vi "Goal Classifier.vi"(5 "ResolutionY":dbl, 7 "ResolutionX":dbl, 11 "InArray":dbl[][](array[numeric])) -> (3 "OutArray":dbl[][](array[numeric]))   [LabVIEW 2012]
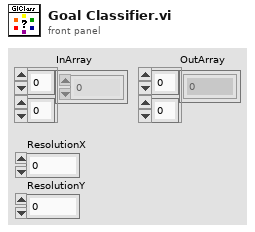
[diagram p1: front panel]
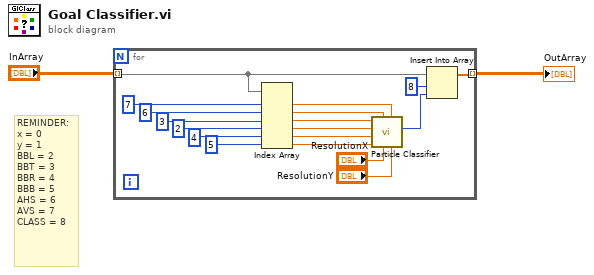
[diagram p0: block diagram]
diagram:
  # "REMINDER:\nx = 0\ny = 1\nBBL = 2\nBBT = 3\nBBR = 4 \nBBB = 5 \nAHS = 6\nAVS = 7 \nCLASS = 8"
  n1 = for {
    tunnel: "InArray" -> [w14] mode=indexing
    tunnel: [w12] -> w1 mode=indexing
    n2 = Index Array(array=w14, index #1=7 ("index"), index #2=6 ("index"), index #3=3 ("index"), index #4=2 ("index"), index #5=4 ("index"), index #6=5 ("index")) -> (element #1=w7:dbl, element #2=w8:dbl, element #3=w6:dbl, element #4=w5:dbl, element #5=w4:dbl, element #6=w3:dbl)
    n3 = call "Particle Classifier.vi"("camResY"="ResolutionY", "vert"=w7, "camResX"="ResolutionX", "horz"=w8, "BndRectBtm"=w3, "BndRectRight"=w4, "BndRectLeft"=w5, "BndRectTop"=w6) -> ("class"=w9:i32)  [unwired: 3 in]
    n4 = Insert Into Array(array=w14, index=8, new element=w9) -> (w12:dbl[])
  }
  "OutArray" <- w1
